vi "List PPLs.vi"(8 "error in":errorcluster) -> (0 "error out":errorcluster, 2 "Loaded?":bool[](array[boolean]), 3 "PPL Details":T1[](array[typedef]))   [LabVIEW 2020, in "ClassLoader.lvlib"]
uses:
  ClassLoader.lvlib
  Ctl/Ctl_PPL Details.ctl
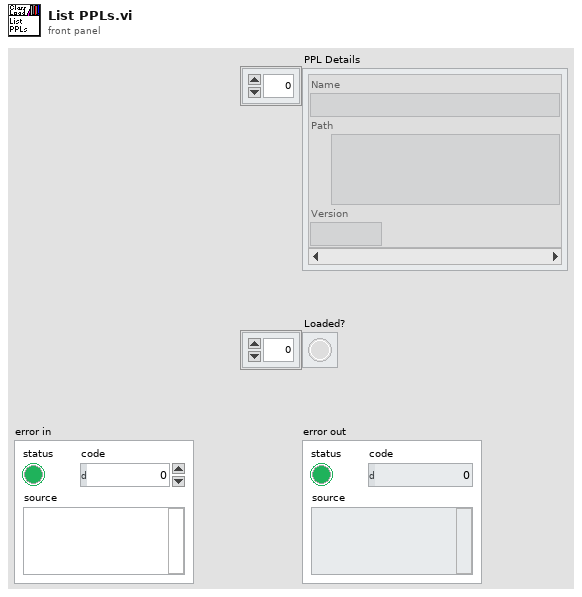
[diagram p1: front panel]
types:
  T1 = typedef "ClassLoader.lvlib/Ctl_PPL Details.ctl" = cluster{"Name":string, "Path":path, "Version":string}
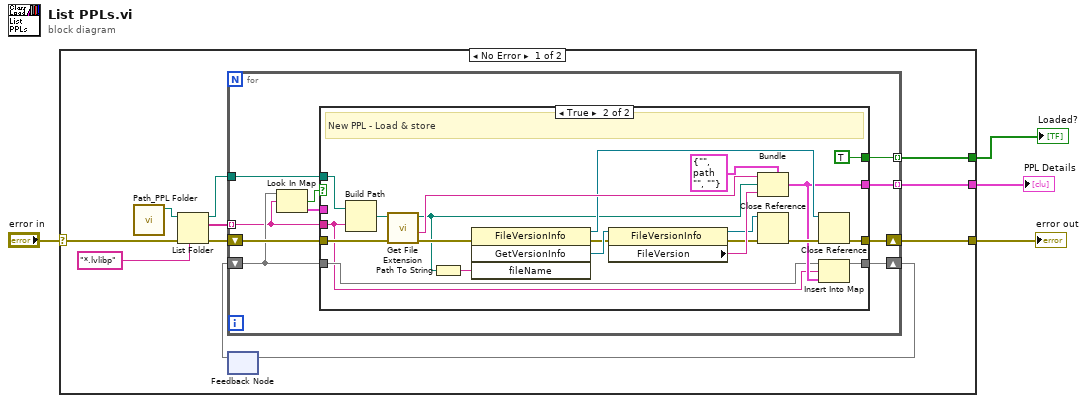
[diagram p0: block diagram]
diagram:
  n1 = case shown="No Error" "error in" {
    selector: "error in" -> [w11 w50]
    tunnel: [w9 w50] -> w3
    tunnel: [w8 _] -> w2
    tunnel: [w5 _] -> w1
    frame No Error {
      n2 = call "Path_PPL Folder.vi"() -> ("Data Folder Path"=w12:path)  [unwired: 10 in, 1 out]
      n3 = List Folder(path=w12, pattern="*.lvlibp", error in=w11) -> (path out=w13:path, filenames=w14:string[], error out=w10:errorcluster)  [unwired: 1 in, 1 out]
      n4 = feedback #1() -> (w6:map{string, T1})  [unwired: 1 in]
      n5 = for {
        tunnel: w14 -> [w19] mode=indexing
        tunnel: w13 -> [w25]
        tunnel: [w22] -> w8 mode=indexing
        shift-right: [w23] -> w9
        shift-left: w10 -> [w24]
        shift-right: [w21] -> w7
        shift-left: w6 -> [w20]
        tunnel: [w16] -> w5 mode=indexing
        n6 = Look In Map(map=w20, key=w19) -> (key not found?=w18:bool, value=w17:T1)  [unwired: 1 in]
        n7 = case shown="True" w18 {
          tunnel: w25 -> [_ w48]
          tunnel: w24 -> [w27 w45]
          tunnel: [w27 w38] -> w23
          tunnel: [w28 w34] -> w22
          tunnel: [w26 w33] -> w21
          tunnel: w20 -> [w26 w31]
          tunnel: w19 -> [_ w30]
          tunnel: w17 -> [w28 _]
          tunnel: [_ TRUE] -> w16
          frame False {
            # "Key found - Return stored data"
          }
          frame True {
            # "New PPL - Load & store"
            n8 = Build Path(base path=w48, name or relative path=w30) -> (appended path=w44:path)
            n9 = call <vilib>:"Get File Extension.vi"("error in (no error)"=w45, "file"=w44) -> ("error out"=w36:errorcluster, "filename without extension"=w43:string, "dup file"=w35:path)  [unwired: 5 in, 2 out]
            n10 = Path To String(path=w35) -> (string=w47:string)
            n11 = invoke class="FileVersionInfo" method="GetVersionInfo"(error in=w36, "fileName"=w47) -> (reference out=w37:refnum<k24>, error out=w42:errorcluster, "GetVersionInfo"=w49:refnum<k24>)  [unwired: 2 in, 1 out]
            n12 = property class="FileVersionInfo"(reference=w49, error in=w42) -> (reference out=w41:refnum<k24>, error out=w40:errorcluster, "FileVersion"=w46:string)
            n13 = Bundle(cluster=T1 {"Name"="", "Path"=path "", "Version"=""}, "Name"=w43, "Path"=w35, "Version"=w46) -> (w34:T1)
            n14 = Close Reference(reference=w41, error in (no error)=w40) -> (error out=w39:errorcluster)
            n15 = Close Reference(reference=w37, error in (no error)=w39) -> (error out=w38:errorcluster)
            n16 = Insert Into Map(map in=w31, key=w30, value=w34) -> (map out=w33:map{string, T1})  [unwired: 2 out]
          }
        }
      }
      n17 = feedback-in #1(w7) -> ()
    }
    frame Error {
    }
  }
  "error out" <- w3
  "PPL Details" <- w2
  "Loaded?" <- w1
